vi "PID_Flow Ctrl_2 P2.vi"(0 "weight":dbl[](array[numeric]), 1 "Setpoint_W":dbl[](array[numeric])=[10.0, 20.0, 30.0], 5 "Setpoint_T":dbl[](array[numeric])=[2.0, 2.0, 2.0], 7 "FrManual":dbl, 8 "enable":i32, 16 "manual":i32, 20 "reset":i32, 24 "tube":i32) -> (2 "elapsed_step":dbl, 3 "total_target":dbl, 4 "Setpoint_W":dbl, 6 "LED_stop":bool, 9 "RPM":dbl, 10 "LED1":bool, 11 "LED4":bool, 12 "LED2":bool, 13 "step_amount":dbl, 14 "LED3":bool, 15 "LED5":bool, 17 "weight":dbl, 19 "time_to_target":dbl, 23 "PumpCTRL":dbl, 25 "step":dbl, 26 "LED_manual":bool, 27 "FR":dbl)   [LabVIEW 2016]
uses:
  BERTTA.dll
panel:
  out "count":dbl
  out "weightChange":dbl
  out "output":dbl
  out "errsum":dbl
  out "error":dbl
  out "setpoint":dbl
  in  "weight":dbl
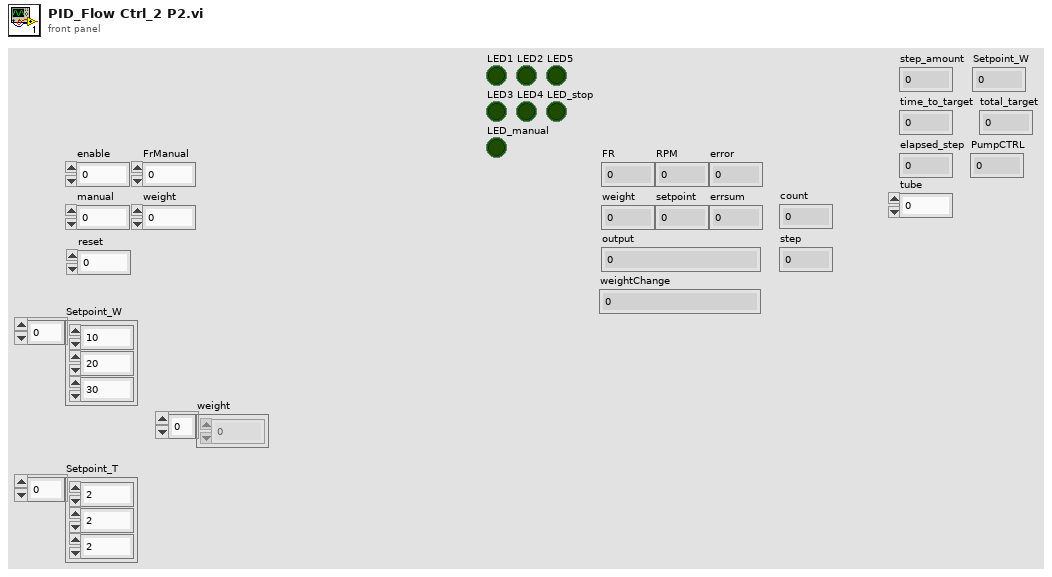
[diagram p1: front panel]
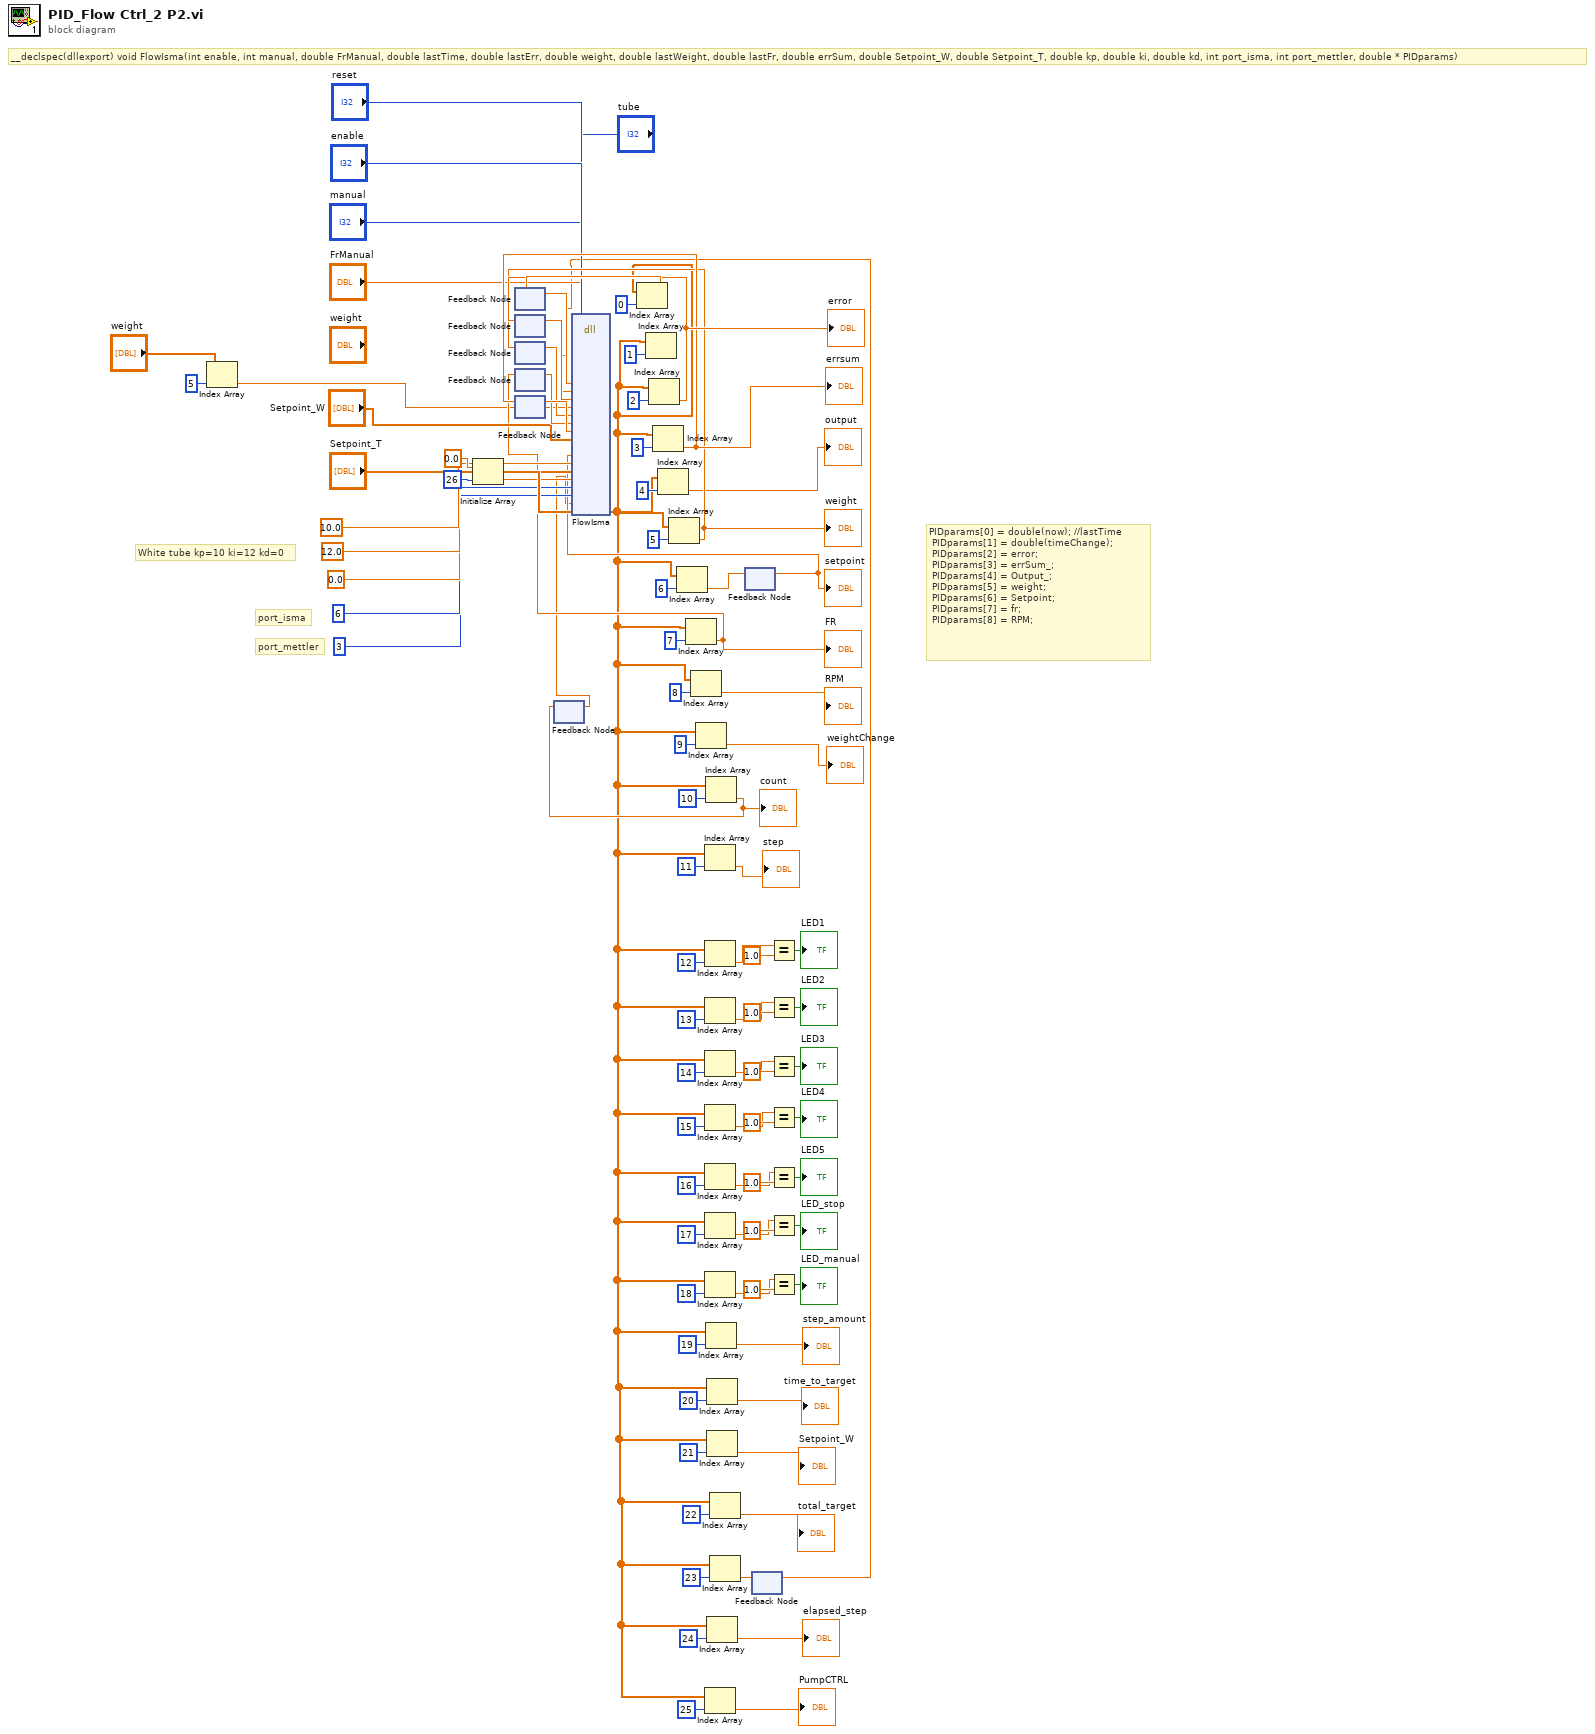
[diagram p0: block diagram]
diagram:
  # "White tube kp=10 ki=12 kd=0"
  # "port_mettler"
  # "port_isma"
  # "PIDparams[0] = double(now); //lastTime \n\tPIDparams[1] = double(timeChange);\n\tPIDparams[2] = error;\n\tPIDparams[3] = errSum_;\n\tPIDparams[4] = Output_;\n\tPIDparams[5] = weight;\n\tPIDparams[6] = Setpoint;\n\tPIDparams[7] = fr;\n\tPIDparams[8] = RPM;"
  # "__declspec(dllexport) void FlowIsma(int enable, int manual, double FrManual, double lastTime, double lastErr, double weight, double lastWeight, double lastFr, double errSum, double Setpoint_W, double Setpoint_T, double kp, double ki, double kd, int port_isma, int port_mettler, double * PIDparams)"
  n1 = Index Array(array="weight", index=5) -> (element=w49:dbl)
  n2 = Initialize Array(0.0 ("element"), 26 ("dimension size")) -> (w90:dbl[])
  n3 = feedback #1() -> (w79:dbl)  [unwired: 1 in]
  n4 = feedback #2() -> (w77:dbl)  [unwired: 1 in]
  n5 = feedback #3() -> (w73:dbl)  [unwired: 1 in]
  n6 = feedback #4() -> (w72:dbl)  [unwired: 1 in]
  n7 = feedback #5() -> (w75:dbl)  [unwired: 1 in]
  n8 = feedback #6() -> (w53:dbl)  [unwired: 1 in]
  n9 = feedback #7() -> (w56:dbl)  [unwired: 1 in]
  "setpoint" <- w56
  n10 = feedback #8() -> (w8:dbl)  [unwired: 1 in]
  n11 = dll-call lib="C:/Users/shresplab/OneDrive - Kemira Oyj/Documents/GitHub/Bertta/BERTTA/x64/Debug/BERTTA.dll" fn="FlowIsma"("reset"="reset", "enable"="enable", "manual"="manual", "tube"="tube", "FrManual"="FrManual", "lastTime"=w79, "elapsed"=w8, "lastErr"=w77, "weight"=w49, "lastWeight"=w73, "lastFr"=w72, "errSum"=w75, "Setpoint_W"="Setpoint_W", "Setpoint_T"="Setpoint_T", "lastSP"=w56, "kp"=10.0, "ki"=12.0, "kd"=0.0, "port_isma"=6, "port_mettler"=3, "count"=w53, "PIDparams"=w90) -> ("PIDparams"=w4:dbl[])  [unwired: 25 in, 2 out]
  n12 = Index Array(array=w4, index=0) -> (element=w80:dbl)
  n13 = feedback-in #1(w80) -> ()
  n14 = Index Array(array=w4, index=1) -> ()  [unwired: 1 out]
  n15 = Index Array(array=w4, index=2) -> (element=w78:dbl)
  "error" <- w78
  n16 = feedback-in #2(w78) -> ()
  n17 = Index Array(array=w4, index=3) -> (element=w76:dbl)
  "errsum" <- w76
  n18 = feedback-in #5(w76) -> ()
  n19 = Index Array(array=w4, index=4) -> (element=→"output":dbl)
  n20 = Index Array(array=w4, index=5) -> (element=w74:dbl)
  "weight" <- w74
  n21 = feedback-in #3(w74) -> ()
  n22 = Index Array(array=w4, index=6) -> (element=w57:dbl)
  n23 = Index Array(array=w4, index=7) -> (element=w58:dbl)
  "FR" <- w58
  n24 = feedback-in #4(w58) -> ()
  n25 = Index Array(array=w4, index=8) -> (element=→"RPM":dbl)
  n26 = Index Array(array=w4, index=9) -> (element=→"weightChange":dbl)
  n27 = Index Array(array=w4, index=11) -> (element=→"step":dbl)
  n28 = Index Array(array=w4, index=12) -> (element=w39:dbl)
  n29 = Index Array(array=w4, index=13) -> (element=w31:dbl)
  n30 = Index Array(array=w4, index=14) -> (element=w30:dbl)
  n31 = Index Array(array=w4, index=15) -> (element=w29:dbl)
  n32 = Index Array(array=w4, index=16) -> (element=w28:dbl)
  n33 = Index Array(array=w4, index=17) -> (element=w27:dbl)
  n34 = Index Array(array=w4, index=18) -> (element=w26:dbl)
  n35 = Index Array(array=w4, index=25) -> (element=→"PumpCTRL":dbl)
  n36 = Index Array(array=w4, index=10) -> (element=w54:dbl)
  "count" <- w54
  n37 = feedback-in #6(w54) -> ()
  n38 = Index Array(array=w4, index=19) -> (element=→"step_amount":dbl)
  n39 = Index Array(array=w4, index=20) -> (element=→"time_to_target":dbl)
  n40 = Index Array(array=w4, index=21) -> (element=→"Setpoint_W":dbl)
  n41 = Index Array(array=w4, index=24) -> (element=→"elapsed_step":dbl)
  n42 = Index Array(array=w4, index=22) -> (element=→"total_target":dbl)
  n43 = Index Array(array=w4, index=23) -> (element=w9:dbl)
  n44 = feedback-in #7(w57) -> ()
  n45 = feedback-in #8(w9) -> ()
  n46 = Equal?(x=w39, y=1.0) -> (x = y?=→"LED1":bool)
  n47 = Equal?(x=w31, y=1.0) -> (x = y?=→"LED2":bool)
  n48 = Equal?(x=w30, y=1.0) -> (x = y?=→"LED3":bool)
  n49 = Equal?(x=w29, y=1.0) -> (x = y?=→"LED4":bool)
  n50 = Equal?(x=w28, y=1.0) -> (x = y?=→"LED5":bool)
  n51 = Equal?(x=w27, y=1.0) -> (x = y?=→"LED_stop":bool)
  n52 = Equal?(x=w26, y=1.0) -> (x = y?=→"LED_manual":bool)
